vi "DAQX mod 1SDI v00.vi"(0 "resource name":refnum<k15>="PXI1Slot2", 1 "close (T)":bool=TRUE, 2 "Record Data":bool, 3 "numSamples":i32=-1, 4 "max time (s)":dbl=10.0 caption="max time", 5 "min sample rate":dbl=100000000.0, 6 "File location":path, 7 "error in":errorcluster, 8 "reference position":dbl=50.0, 10 "Type of\nmeasurement":T1, 11 "Name root":string, 13 "channel parameters":T3(array[cluster])=[{"channel name"="0", "input impedance"=0, "maximum input frequency"=30000000.0, "vertical coupling"=1, "probe attenuation"=1.0, "vertical range"=2.0, "vertical offset"=0.0, "channel enabled"=TRUE}, {"channel name"="1", "input impedance"=0, "maximum input frequency"=30000000.0, "vertical coupling"=1, "probe attenuation"=1.0, "vertical range"=2.0, "vertical offset"=0.0, "channel enabled"=TRUE}] {"input impedance" items=["1 mega ohm"=0, "50 ohms"=2]; "vertical coupling" items=["AC", "DC", "Ground"]}, 15 "reset sn":bool) -> (18 "wfm out":waveform(dbl)[](array[waveform]), 22 "Parameters values file":string, 24 "actualSamples 0":i32, 26 "actualSamples 1":i32, 27 "error out":errorcluster caption="error out final")   [LabVIEW 2013]
doc: "Configures and acquires data from an NI-SCOPE high-speed digitizer.\n--------------------\n\nThis Express VI is configured as follows:\n\nDevice: PXI1Slot2 (PXI-5122)\nSample Rate (S/s): 100M\nRecord length: 2k\nAcquisition Mode: N Samples\nChannel 0\n - Range (V): 2\n - Offset (V): 0\n - Probe attenuation: 1\n - Coupling: \n - Input impedence: 1 \n - Bandwidth (Hz): 0\nChannel 1\n - Range (V): 2\n - Offset (V): 0\n - Probe attenuation: 1\n - Coupling: \n - Input impedence: 1 \n - Bandwidth (Hz): 0\nImmediate"
uses:
  <instrlib>/niScope/Controls/niScope vertical coupling.ctl
  Strict Type Defs/type_meas_enum.ctl
  <instrlib>/niScope/Controls/niScope timestamp type.ctl
  <instrlib>/niScope/Acquire/Fetch/niScope Multi Fetch Binary 16.vi
  <instrlib>/niScope/Acquire/Fetch/niScope Multi Fetch WDT.vi
  <instrlib>/niScope/Configure/Trigger/niScope Configure Trigger Immediate.vi
  Global VIs/shotnoise.vi
panel:
  out "gain 1":dbl
  out "offset 1":dbl
  out "xIncrement 1":dbl
  out "relativeInitialX 1":dbl
  out "file location into parameter files":path
  out "size(s)":i32
  out "gain 0":dbl
  out "offset 0":dbl
  out "xIncrement 0":dbl
  out "relativeInitialX 0":dbl
  out "actual sample rate":dbl
  in  "Additional text":string
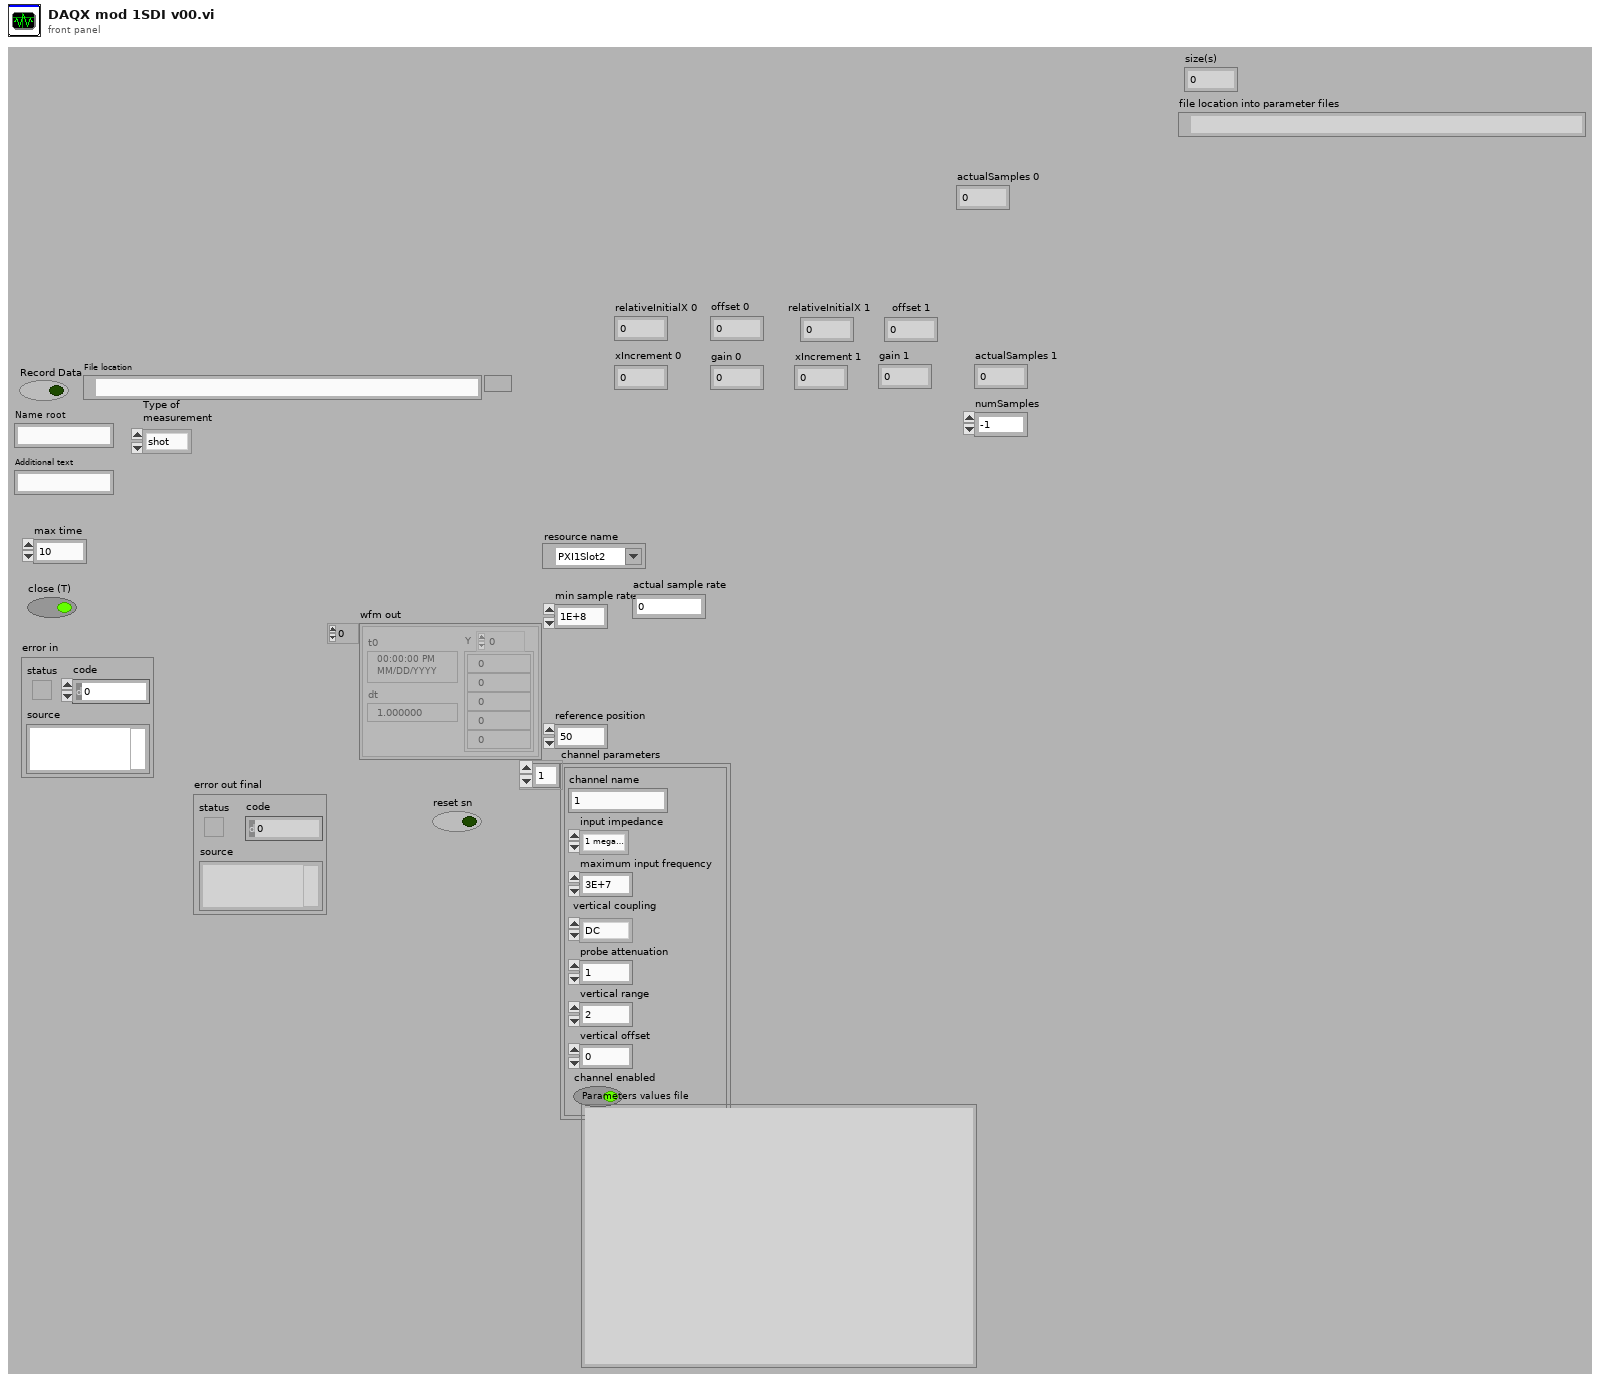
[diagram p1: front panel]
types:
  T1 = typedef "type_meas_enum.ctl" = enum16{"shot", "x", "p", "electronic"}
  T2 = typedef "niScope vertical coupling.ctl" = i32
  T3 = cluster{"channel name":string, "input impedance":u32, "maximum input frequency":dbl, "vertical coupling":T2, "probe attenuation":dbl, "vertical range":dbl, "vertical offset":dbl, "channel enabled":bool}[]
  T4 = typedef "niScope timestamp type.ctl" = i32
  T5 = cluster{"actualSamples":i32, "absoluteInitialX":dbl, "relativeInitialX":dbl, "xIncrement":dbl, "offset":dbl, "gain":dbl, "reserved1":dbl, "reserved2":dbl}[]
  T6 = cluster{"actualSamples":i32, "absoluteInitialX":dbl, "relativeInitialX":dbl, "xIncrement":dbl, "offset":dbl, "gain":dbl, "reserved1":dbl, "reserved2":dbl}
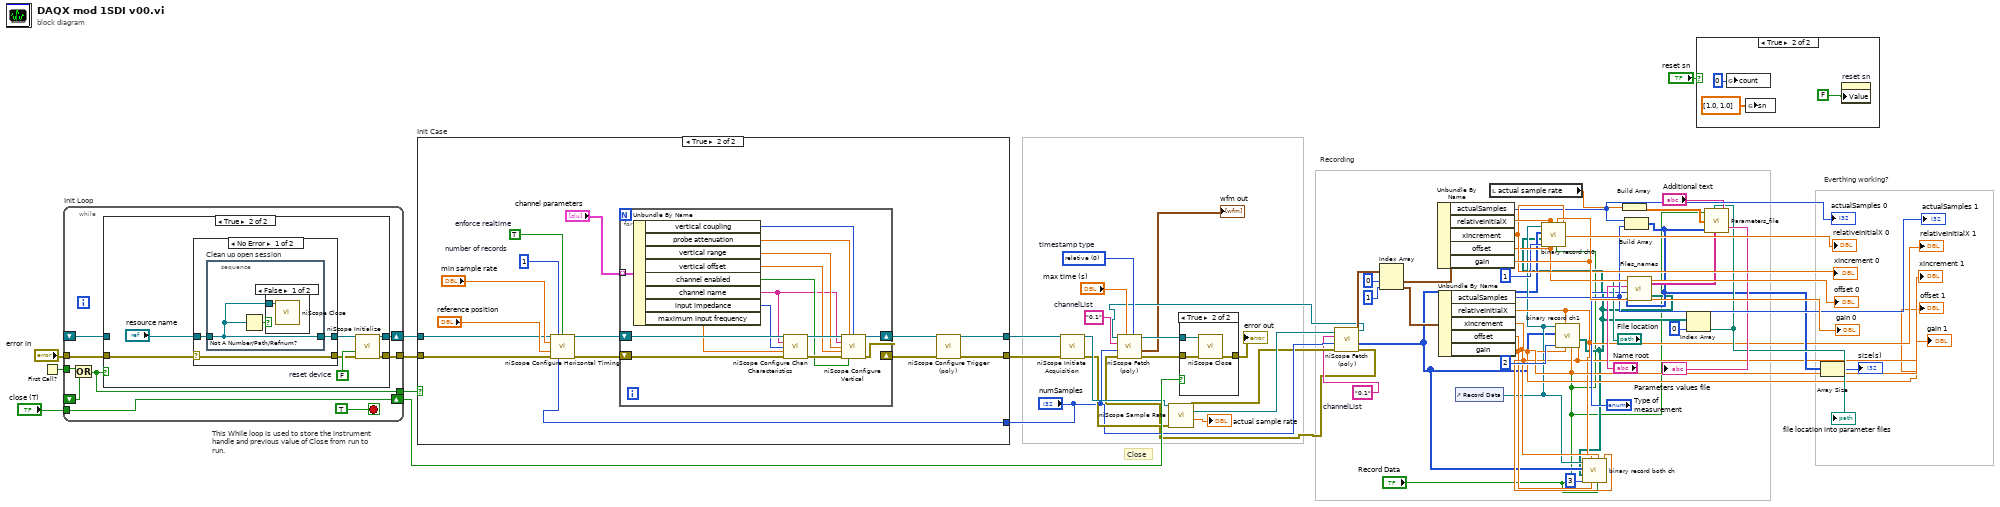
[diagram p0: block diagram]
diagram:
  w14 = "0,1"  # channelList
  w55 = T4 0 items=["relative", "absolute"]  # timestamp type
  w58 = "0,1"  # channelList
  # "Everthing working?"
  # "Recording"
  # "This While loop is used to store the instrument handle and previous value of Close from run to run."
  # "Close"
  n1 = First Call?() -> (First Call?: T/F=w54:bool)
  n2 = while "Init Loop" {
    tunnel: w54 -> [w69]
    shift-right: [w68] -> w50
    shift-left: _ -> [w65]
    tunnel: "close (T)" -> [w68]
    shift-right: [w67] -> w53
    shift-left: _ -> [w66]
    tunnel: [w63] -> w52
    tunnel: "error in" -> [w62]
    tunnel: [w61] -> w51
    stop <- TRUE ("stopInit") stop-if-true
    n3 = Or(x=w69, y=w65) -> (x .or. y?=w61:bool)
    n4 = case "Select_Init" shown="True" w61 {
      tunnel: [w71 w76] -> w67
      tunnel: w66 -> [w71 _]
      tunnel: [w70 w75] -> w63
      tunnel: w62 -> [w70 w74]
      frame False {
      }
      frame True {
        w77 = FALSE  # reset device
        n5 = case shown="No Error" w74 {
          selector: w74 -> [w79 w85]
          tunnel: [w81 w86] -> w78
          tunnel: "resource name" -> [w80 w86]
          tunnel: [w79 w85] -> w73
          frame No Error {
            n6 = stacked-sequence "Clean up open session" {
              tunnel: w80 -> [w82]
              tunnel: [w82] -> w81
              frame #0 {
                n7 = Not A Number/Path/Refnum?(number/path/refnum=w82) -> (NaN/Path/Refnum?=w83:bool)
                n8 = case shown="False" w83 {
                  tunnel: w82 -> [w84 _]
                  frame False {
                    n9 = call <instrlib>:"niScope Close.vi"("instrument handle"=w84) -> ()  [unwired: 1 in, 14 out]
                  }
                  frame True {
                  }
                }
              }
            }
          }
          frame Error {
          }
        }
        n10 = call <instrlib>:"niScope Initialize.vi"("resource name"=w78, "reset device"=w77, "error in"=w73) -> ("instrument handle"=w76:refnum<k15>, "error out"=w75:errorcluster)  [unwired: 2 in, 9 out]
      }
    }
  }
  n11 = case "Init Case" shown="True" w51 {
    tunnel: w52 -> [w87 w93]
    tunnel: [w87 w95] -> w57
    tunnel: [w88 w96] -> w56
    tunnel: w53 -> [w88 w94]
    tunnel: "numSamples" -> [_ w89]
    frame False {
    }
    frame True {
      w101 = 1  # number of records
      w102 = TRUE  # enforce realtime
      n12 = call <instrlib>:"niScope Configure Horizontal Timing.vi"("instrument handle"=w94, "number of records"=w101, "enforce realtime"=w102, "min sample rate"="min sample rate", "reference position"="reference position", "error in"=w93, "min record length"=w89) -> ("instrument handle out"=w97:refnum<k15>, "error out"=w98:errorcluster)  [unwired: 7 out]
      n13 = for {
        shift-right: [w105] -> w90
        shift-left: w98 -> [w117]
        shift-right: [w104] -> w91
        shift-left: w97 -> [w116]
        tunnel: "channel parameters" -> [w113] mode=indexing
        n14 = Unbundle By Name(w113) -> ("vertical coupling"=w110:T2, "probe attenuation"=w109:dbl, "vertical range"=w108:dbl, "vertical offset"=w107:dbl, "channel enabled"=w106:bool, "channel name"=w103:string, "input impedance"=w111:u32, "maximum input frequency"=w112:dbl)
        n15 = call <instrlib>:"niScope Configure Chan Characteristics.vi"("instrument handle"=w116, "channels"=w103, "input impedance"=w111, "maximum input frequency"=w112, "error in"=w117) -> ("instrument handle out"=w115:refnum<k15>, "error out"=w114:errorcluster)  [unwired: 9 out]
        n16 = call <instrlib>:"niScope Configure Vertical.vi"("instrument handle"=w115, "probe attenuation"=w109, "vertical coupling"=w110, "channels"=w103, "vertical range"=w108, "vertical offset"=w107, "error in"=w114, "channel enabled"=w106) -> ("instrument handle out"=w104:refnum<k15>, "error out"=w105:errorcluster)  [unwired: 6 out]
      }
      n17 = call-poly <instrlib>:"niScope Configure Trigger (poly).vi"("instrument handle"=w91, "error in"=w90) -> ("instrument handle out"=w96:refnum<k15>, "error out"=w95:errorcluster)  [unwired: 12 out]
    }
  }
  n18 = call <instrlib>:"niScope Initiate Acquisition.vi"("instrument handle"=w56, "error in"=w57) -> ("instrument handle out"=w46:refnum<k15>, "error out"=w45:errorcluster)  [unwired: 12 out]
  n19 = call <instrlib>:"niScope Sample Rate.vi"("instrument handle"=w46, "error in"=w45) -> ("instrument handle out"=w41:refnum<k15>, "actual sample rate"=→"actual sample rate":dbl, "error out"=w40:errorcluster)  [unwired: 11 out]
  n20 = call-poly <instrlib>:"niScope Fetch (poly).vi"("error in"=w40, "numSamples"="numSamples", "channels"=w14, "instrument handle"=w41) -> ("error out"=w7:errorcluster, "wfm"=w5:i16[][], "wfm info"=w39:T5, "instrument handle out"=w8:refnum<k15>)  [unwired: 1 in, 3 out]
  n21 = call-poly <instrlib>:"niScope Fetch (poly).vi"("timestamp Type"=w55, "timeout"="max time (s)", "error in"=w7, "numSamples"="numSamples", "channels"=w58, "instrument handle"=w8) -> ("error out"=w2:errorcluster, "wfm"=→"wfm out":waveform(dbl)[], "instrument handle out"=w44:refnum<k15>)  [unwired: 3 out]
  n22 = case shown="True" w50 {
    tunnel: w2 -> [w118 w121]
    tunnel: [w118 w120] -> w60
    tunnel: w44 -> [_ w119]
    frame False {
    }
    frame True {
      n23 = call <instrlib>:"niScope Close.vi"("instrument handle"=w119, "error in"=w121) -> ("error out"=w120:errorcluster)  [unwired: 13 out]
    }
  }
  "error out" <- w60
  n24 = Index Array(array=w39, index #1=0 ("index"), index #2=1 ("index")) -> (element #1=w36:T6, element #2=w35:T6)
  n25 = Unbundle By Name(w36) -> ("actualSamples"=w28:i32, "relativeInitialX"=w34:dbl, "xIncrement"=w32:dbl, "offset"=w31:dbl, "gain"=w33:dbl)
  "actualSamples 0" <- w28
  "relativeInitialX 0" <- w34
  "xIncrement 0" <- w32
  "offset 0" <- w31
  "gain 0" <- w33
  n26 = Unbundle By Name(w35) -> ("actualSamples"=w27:i32, "relativeInitialX"=w11:dbl, "xIncrement"=w12:dbl, "offset"=w10:dbl, "gain"=w13:dbl)
  "actualSamples 1" <- w27
  "relativeInitialX 1" <- w11
  "xIncrement 1" <- w12
  "offset 1" <- w10
  "gain 1" <- w13
  n27 = control-ref of="Record Data"() -> (w6:refnum<vi>)
  n28 = local read "actual sample rate"() -> (w18:dbl)
  n29 = Build Array(w18) -> (w17:dbl[])
  n30 = Build Array(w28, w27) -> (w16:i32[])
  n31 = call "Files_names.vi"("actualSamples\narray"=w16, "Type of\nmeasurement"="Type of\nmeasurement", "Name root"="Name root", "File location"="File location") -> ("Files path array"=w4:path[], "Files name array"=w23:string[])
  n32 = call "binary record ch0.vi"("xIncrement"=w32, "Record"="Record Data", "gain"=w33, "offset"=w31, "relativeInitialX"=w34, "Index files\npath array"=1 ("Index files\npath array"), "Files path array"=w4, "wfm"=w5, "reference"=w6) -> ()  [unwired: 3 out]
  n33 = call "binary record ch1.vi"("xIncrement"=w12, "Record"="Record Data", "gain"=w13, "offset"=w10, "relativeInitialX"=w11, "Index files\npath array"=2 ("Index files\npath array"), "Files path array"=w4, "wfm"=w5, "reference"=w6) -> ()  [unwired: 3 out]
  n34 = call "binary record both ch.vi"("xIncrement"=w12, "Record"="Record Data", "gain"=w13, "offset"=w10, "relativeInitialX"=w11, "Index files\npath array"=3 ("Index files\npath array"), "Files path array"=w4, "wfm"=w5, "reference"=w6) -> ()  [unwired: 3 out]
  n35 = Index Array(array=w4, index=0) -> (element=w20:path)
  "file location into parameter files" <- w20
  n36 = case shown="True" "reset sn" {
    frame False {
    }
    frame True {
      n37 = global write "shotnoise.vi" "count"(i64 0 ("count")) -> ()
      n38 = global write "shotnoise.vi" "sn"(dbl[] [1.0, 1.0] ("sn")) -> ()
      n39 = property on="reset sn" class="Bool (strict)"("Value"=FALSE ("reset sn")) -> ()  [unwired: 2 in, 2 out]
    }
  }
  n40 = call "Parameters_file.vi"("Record"="Record Data", "File location"=w20, "actual sample rate array"=w17, "actualSamples array"=w16, "Files name array"=w23, "Additional text"="Additional text") -> ("Full text"=→"Parameters values file":string)
  n41 = Array Size(array=w16) -> (size(s)=→"size(s)":i32)
